vi "ReadAcquisitionSettings.vi"(8 "error in (no error)":errorcluster, 11 "Map":T1) -> (0 "error out":errorcluster, 1 "OSClkStart":dbl, 3 "Running Acquisition Length":dbl, 4 "Acquisition Block Number":i32, 5 "Block Size (s)":dbl, 7 "dt":dbl)   [LabVIEW 2017]
uses:
  <vilib>/addons/PointValueMap/controls/PointMap.ctl
  <vilib>/addons/PointValueMap/subVIs/Point_Read_double.vi
  <vilib>/addons/PointValueMap/subVIs/Point_Read_i32.vi
  <vilib>/addons/PointValueMap/PointValueMap.lvlib
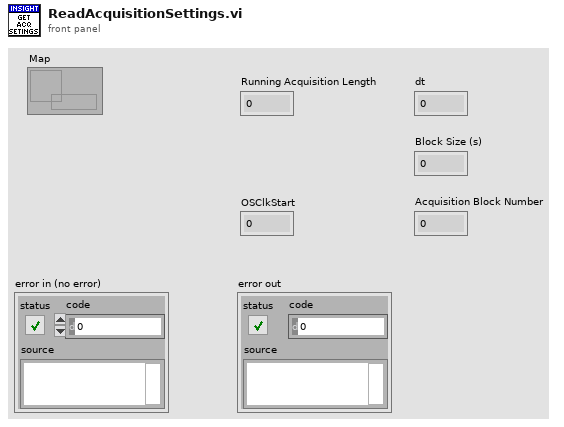
[diagram p1: front panel]
types:
  T1 = typedef "PointValueMap.lvlib/PointMap.ctl" = refnum<data-value>
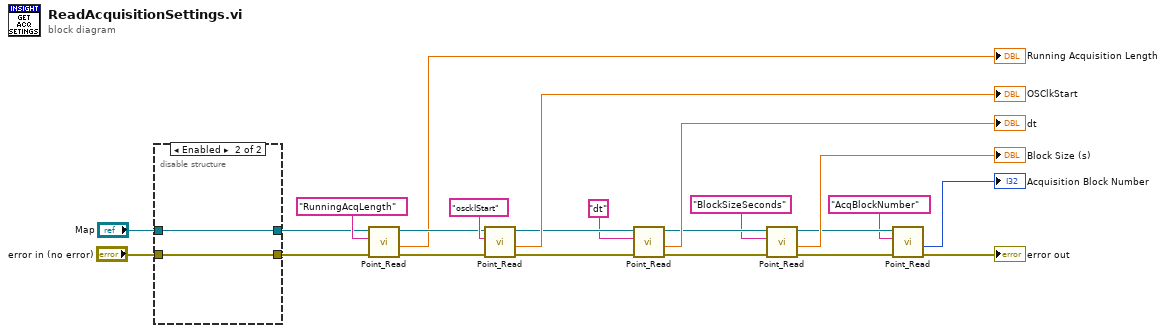
[diagram p0: block diagram]
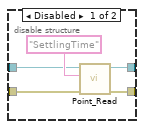
[diagram p2: hidden frame]
diagram:
  n1 = disable-structure shown="Enabled" {
    disable-tunnel: "Map" -> [w27 w30]
    disable-tunnel: [w26 w30] -> w16
    disable-tunnel: [w25 w29] -> w15
    disable-tunnel: "error in (no error)" -> [w24 w29]
    frame Disabled {
      n2 = call-poly <vilib>:"Point_Read.vi"("Error In"=w24, "Tag"="SettlingTime", "Map"=w27) -> ("Error Out"=w25:errorcluster, "Map Out"=w26:T1)  [unwired: 3 in, 4 out]
    }
    frame Enabled {
    }
  }
  n3 = call-poly <vilib>:"Point_Read.vi"("Error In"=w15, "Tag"="RunningAcqLength", "Map"=w16) -> ("Error Out"=w18:errorcluster, "Value"=→"Running Acquisition Length":dbl, "Map Out"=w21:T1)  [unwired: 3 in, 3 out]
  n4 = call-poly <vilib>:"Point_Read.vi"("Error In"=w18, "Tag"="oscklStart", "Map"=w21) -> ("Error Out"=w12:errorcluster, "Value"=→"OSClkStart":dbl, "Map Out"=w13:T1)  [unwired: 3 in, 3 out]
  n5 = call-poly <vilib>:"Point_Read.vi"("Error In"=w12, "Tag"="dt", "Map"=w13) -> ("Error Out"=w8:errorcluster, "Value"=→"dt":dbl, "Map Out"=w9:T1)  [unwired: 3 in, 3 out]
  n6 = call-poly <vilib>:"Point_Read.vi"("Error In"=w8, "Tag"="BlockSizeSeconds", "Map"=w9) -> ("Error Out"=w3:errorcluster, "Value"=→"Block Size (s)":dbl, "Map Out"=w5:T1)  [unwired: 3 in, 3 out]
  n7 = call-poly <vilib>:"Point_Read.vi"("Error In"=w3, "Tag"="AcqBlockNumber", "Map"=w5) -> ("Error Out"=→"error out":errorcluster, "Value"=→"Acquisition Block Number":i32)  [unwired: 3 in, 4 out]
